vi "Fetch Multi Eval Meas List ES Flatness Results.vi"(7 "Result Type (Current)":i32(ring) items=["Current", "Average", "Extreme", "Standard Deviation"], 8 "error in (no error)":errorcluster, 9 "Difference (Difference 1)":T1=1 items=["Difference 1"=1, "Difference 2"=2], 10 "Instance (1)":T2=1, 11 "VISA resource name":refnum<visa-resource-name>) -> (0 "error out":errorcluster, 1 "ES Flatness Results":dbl[](array[numeric]) format="%^.3e", 2 "Reliability":i32, 3 "VISA resource name out":refnum<visa-resource-name>)   [LabVIEW 2015, in "Rohde&Schwarz CMXP NR FR2 Measurement.lvlib"]
doc: "Returns equalizer spectrum flatness single value results (differences between ranges) for all measured list mode segments.\n\nAttributes:\nRSCMXPNRFR2M_ATTR_FETCH_MULTI_EVAL_MEASUREMENT_LIST_ESF_AVERAGE_RESULTS\nRSCMXPNRFR2M_ATTR_FETCH_MULTI_EVAL_MEASUREMENT_LIST_ESF_CURRENT_RESULTS\nRSCMXPNRFR2M_ATTR_FETCH_MULTI_EVAL_MEASUREMENT_LIST_ESF_EXTREME_RESULTS\nRSCMXPNRFR2M_ATTR_FETCH_MULTI_EVAL_MEASUREMENT_LIST_ESF_STANDARD_DEVIATION_RESULTS\n\nRemote-control commands:\nFETCh:NRMMw:MEAS<i>:MEValuation:LIST:ESFLatness:DIFFerence<no>:AVERage?\nFETCh:NRMMw:MEAS<i>:MEValuation:LIST:ESFLatness:DIFFerence<no>:CURRent?\nFETCh:NRMMw:MEAS<i>:MEValuation:LIST:ESFLatness:DIFFerence<no>:EXTReme?\nFETCh:NRMMw:MEAS<i>:MEValuation:LIST:ESFLatness:DIFFerence<no>:SDEViation?"
uses:
  <instrlib>/Rohde&Schwarz CMXP NR FR2 Measurement/Rohde&Schwarz CMXP NR FR2 Measurement.lvlib
  <instrlib>/Rohde&Schwarz CMXP NR FR2 Measurement/Private/_Instance.ctl
  <instrlib>/Rohde&Schwarz CMXP NR FR2 Measurement/Private/_Difference.ctl
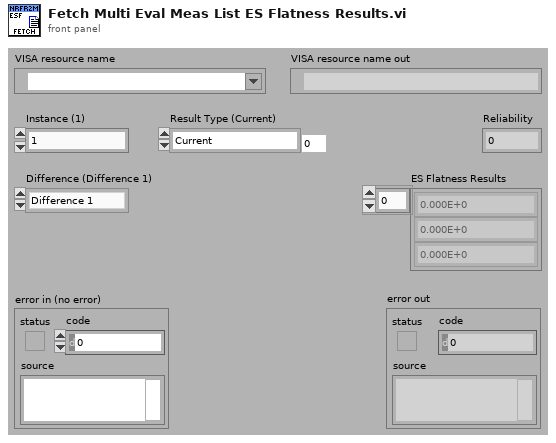
[diagram p1: front panel]
types:
  T1 = typedef "Rohde&Schwarz CMXP NR FR2 Measurement.lvlib/_Difference.ctl" = i32
  T2 = typedef "Rohde&Schwarz CMXP NR FR2 Measurement.lvlib/_Instance.ctl" = i32
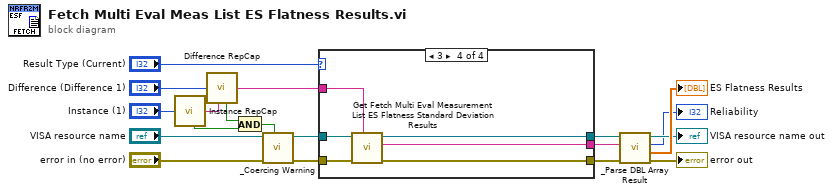
[diagram p0: block diagram]
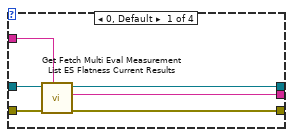
[diagram p2: hidden frame]
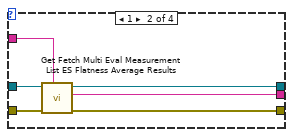
[diagram p3: hidden frame]
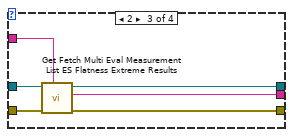
[diagram p4: hidden frame]
diagram:
  n1 = call <instrlib>:"Instance RepCap.vi"("Instance In"="Instance (1)") -> ("In Range?"=w15:bool, "RepCap Identifier Out"=w1:string)  [unwired: 1 in]
  n2 = call <instrlib>:"Difference RepCap.vi"("Difference In"="Difference (Difference 1)", "RepCap String In (\"\")"=w1) -> ("In Range?"=w16:bool, "RepCap Identifier Out"=w13:string)
  n3 = And(x=w16, y=w15) -> (x .and. y?=w18:bool)
  n4 = call <instrlib>:"_Coercing Warning.vi"("In Range?"=w18, "error in (no error)"="error in (no error)", "VISA resource name"="VISA resource name") -> ("error out"=w11:errorcluster, "VISA resource name out"=w12:refnum<visa-resource-name>)  [unwired: 7 in]
  n5 = case shown="3" "Result Type (Current)" {
    tunnel: w13 -> [w25 w31 w37 w43]
    tunnel: w12 -> [w24 w30 w36 w42]
    tunnel: w11 -> [w23 w29 w35 w41]
    tunnel: [w22 w28 w34 w40] -> w9
    tunnel: [w21 w27 w33 w39] -> w7
    tunnel: [w20 w26 w32 w38] -> w8
    frame 0, Default {
      n6 = call "Get Fetch Multi Eval Measurement List ES Flatness Current Results"("Repeated Capabilities"=w25, "error in (no error)"=w23, "instrument handle"=w24) -> ("error out"=w22:errorcluster, "Fetch Multi Eval Measurement List ES Flatness Current Results"=w20:string, "instrument handle out"=w21:refnum<visa-resource-name>)  [unwired: 6 in]
    }
    frame 1 {
      n7 = call "Get Fetch Multi Eval Measurement List ES Flatness Average Results"("Repeated Capabilities"=w31, "error in (no error)"=w29, "instrument handle"=w30) -> ("error out"=w28:errorcluster, "Fetch Multi Eval Measurement List ES Flatness Average Results"=w26:string, "instrument handle out"=w27:refnum<visa-resource-name>)  [unwired: 6 in]
    }
    frame 2 {
      n8 = call "Get Fetch Multi Eval Measurement List ES Flatness Extreme Results"("Repeated Capabilities"=w37, "error in (no error)"=w35, "instrument handle"=w36) -> ("error out"=w34:errorcluster, "Fetch Multi Eval Measurement List ES Flatness Extreme Results"=w32:string, "instrument handle out"=w33:refnum<visa-resource-name>)  [unwired: 6 in]
    }
    frame 3 {
      n9 = call "Get Fetch Multi Eval Measurement List ES Flatness Standard Deviation Results"("Repeated Capabilities"=w43, "error in (no error)"=w41, "instrument handle"=w42) -> ("error out"=w40:errorcluster, "Fetch Multi Eval Measurement List ES Flatness Standard Deviation Results"=w38:string, "instrument handle out"=w39:refnum<visa-resource-name>)  [unwired: 6 in]
    }
  }
  n10 = call <instrlib>:"_Parse DBL Array Result.vi"("error in (no error)"=w9, "Input String"=w8, "VISA resource name"=w7) -> ("error out"=→"error out":errorcluster, "Results"=→"ES Flatness Results":dbl[], "Reliability"=→"Reliability":i32, "VISA resource name out"=→"VISA resource name out":refnum<visa-resource-name>)  [unwired: 5 in]
